vi "Ball-Goal Impact.vi"(9 "Field Length":dbl, 10 "Ball":T1, 11 "Ball Velocity":dbl[](array[numeric])) -> (3 "Y Collision":dbl)   [LabVIEW 2016]
uses:
  Core/AI Ball.ctl
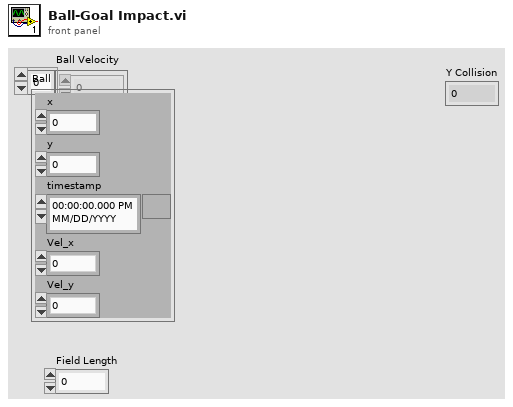
[diagram p1: front panel]
types:
  T1 = typedef "AI Ball.ctl" = cluster{"x":dbl, "y":dbl, "timestamp":timestamp, "Vel_x":dbl, "Vel_y":dbl}
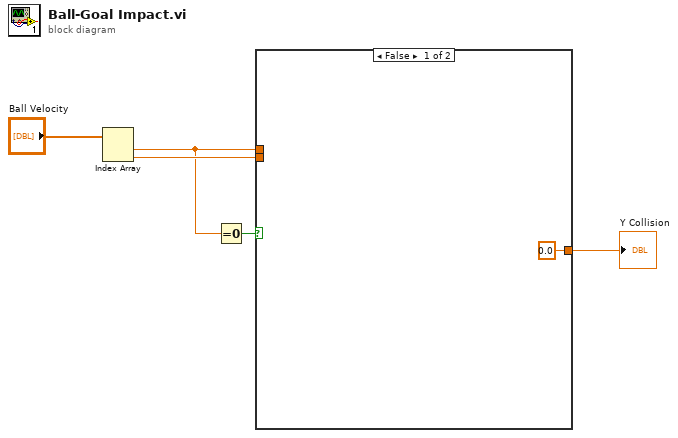
[diagram p0: block diagram]
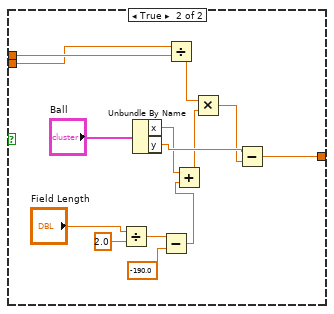
[diagram p2: hidden frame]
diagram:
  n1 = Index Array(array="Ball Velocity") -> (element #1=w1:dbl, element #2=w4:dbl)  [unwired: 2 in]
  n2 = Equal To 0?(x=w1) -> (x = 0?=w2:bool)
  n3 = case shown="False" w2 {
    tunnel: w1 -> [_ w18]
    tunnel: w4 -> [_ w17]
    tunnel: [0.0 w14] -> w3
    frame False {
    }
    frame True {
      n4 = Divide(x="Field Length", y=2.0) -> (x/y=w9:dbl)
      n5 = Unbundle By Name("Ball") -> ("x"=w13:dbl, "y"=w19:dbl)
      n6 = Subtract(x=w9, y=-190.0) -> (x-y=w7:dbl)
      n7 = Divide(x=w17, y=w18) -> (x/y=w16:dbl)
      n8 = Add(x=w13, y=w7) -> (x+y=w12:dbl)
      n9 = Multiply(x=w16, y=w12) -> (x*y=w15:dbl)
      n10 = Subtract(x=w19, y=w15) -> (x-y=w14:dbl)
    }
  }
  "Y Collision" <- w3
